vi "Test_Caraya_Example.vi"() -> ()   [LabVIEW 2013]
uses:
  <vilib>/addons/_JKI Toolkits/Caraya/classes/Assert/Assert True.vi
  <vilib>/addons/_JKI Toolkits/Caraya/classes/Test/Test.lvclass
  <vilib>/addons/_JKI Toolkits/Caraya/classes/Assert/Assert.lvclass
panel:
  in  "error in (no error)":errorcluster
  out "error out":errorcluster
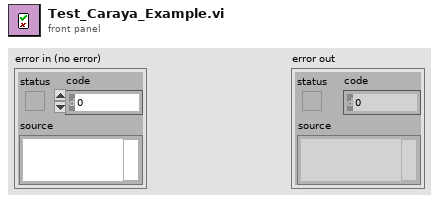
[diagram p1: front panel]
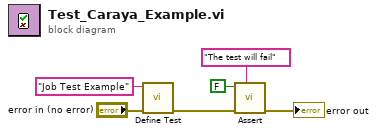
[diagram p0: block diagram]
diagram:
  n1 = call <vilib>:"Define Test.vi"("error in (no error)"="error in (no error)", "Label (VI Title)"="Job Test Example") -> ("error out"=w6:errorcluster)  [unwired: 9 in]
  n2 = call-poly <vilib>:"Assert.vi"("Label"="The test will fail" ("Label (VI Title)"), "error in (no error)"=w6, "True?"=FALSE) -> ("error out"=→"error out":errorcluster)  [unwired: 8 in]
